vi "create channels from PID element.vi"(11 "line item in":T1) -> (1 "Output Channel Out":refnum<class "TBM channel.lvclass">, 2 "Process Variable Channel Out":refnum<class "TBM channel.lvclass">, 3 "Setpoint Channel Out":refnum<class "TBM channel.lvclass">)   [LabVIEW 2015, in "PID Module configuration.lvclass"]
uses:
  module/configuration/PID Module configuration.lvclass
  <vilib>/NI/Tag Bus Module Framework/channel/TBM channel.lvclass
  PID array element.ctl
  <vilib>/NI/Tag Bus Module Framework/channel/channel classification.ctl
  <vilib>/NI/Tag Bus/tag/Data Type.ctl
  <vilib>/NI/Tag Bus/tag/tag descriptor.lvclass
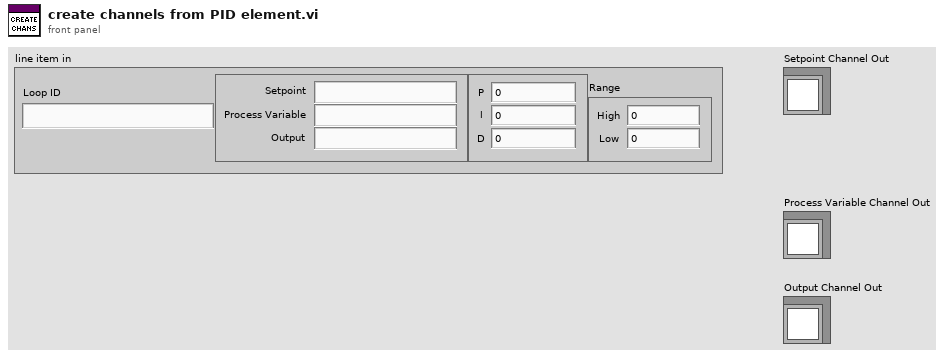
[diagram p1: front panel]
types:
  T1 = typedef "PID Module configuration.lvclass/PID array element.ctl" = cluster{"Loop ID":string, "Tags":cluster{"Setpoint":string, "Process Variable":string, "Output":string}, "Gains":cluster{"P":dbl, "I":dbl, "D":dbl}, "Range":cluster{"High":dbl, "Low":dbl}}
  T2 = typedef "tag bus.lvlib/tag descriptor.lvclass/Data Type.ctl" = enum16{"Double", "Single", "I64", "I32", "I16", "I8", "U64", "U32", "U16", "U8", "Boolean", "String", "Array of Double", "Array of Single", "Array of I64", "Array of I32", "Array of I16", "Array of I8", "Array of U64", "Array of U32", "Array of U16", "Array of U8", "Array of Boolean", "Array of String"}
  T3 = typedef "TBM channel.lvclass/channel classification.ctl" = enum16{"input data", "output data", "processing parameter", "processing result"}
  T4 = cluster{"Setpoint Channel":string, "Process Variable Channel":string, "Output Channel":string}
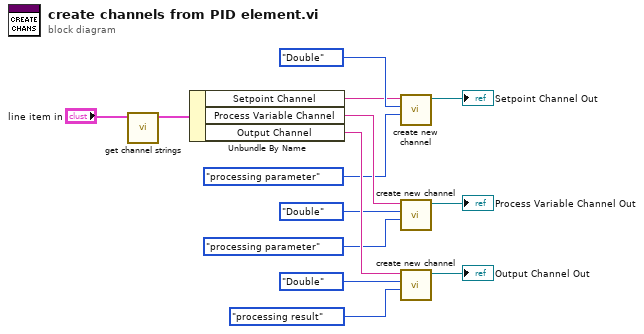
[diagram p0: block diagram]
diagram:
  n1 = call "get channel strings.vi"("line item in"="line item in") -> ("Tag Names"=w2:T4)  [unwired: 10 in]
  n2 = Unbundle By Name(w2) -> ("Setpoint Channel"=w3:string, "Process Variable Channel"=w10:string, "Output Channel"=w11:string)
  n3 = call <vilib>:"create new channel.vi"("channel classification"=channel_classification."processing parameter", "data type"=Data_Type."Double", "channel name"=w3) -> ("channel"=→"Setpoint Channel Out":refnum<class "TBM channel.lvclass">)  [unwired: 8 in]
  n4 = call <vilib>:"create new channel.vi"("channel classification"=channel_classification."processing parameter", "data type"=Data_Type."Double", "channel name"=w10) -> ("channel"=→"Process Variable Channel Out":refnum<class "TBM channel.lvclass">)  [unwired: 8 in]
  n5 = call <vilib>:"create new channel.vi"("channel classification"=channel_classification."processing result", "data type"=Data_Type."Double", "channel name"=w11) -> ("channel"=→"Output Channel Out":refnum<class "TBM channel.lvclass">)  [unwired: 8 in]
